vi "Sound-Beeper.vi"() -> (15 "error out":errorcluster)   [LabVIEW 2020]
uses:
  <vilib>/sound2/lvsound2.llb/Sampling Mode.ctl
  <vilib>/sound2/lvsound2.llb/Sound Data Format.ctl
  Math VIs/LinSpace (x0-dx-npts).vi
  <vilib>/sound2/lvsound2.llb/Sound Output Write (DBL Single).vi
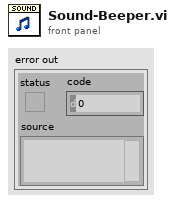
[diagram p1: front panel]
types:
  T1 = typedef "Sound Data Format.ctl" = cluster{"sample rate (S/s)":dbl, "number of channels":i32, "bits per sample":i32}
  T2 = typedef "Sampling Mode.ctl" = i32
  T3 = typedef "Sound Output Task ID.ctl" = u32
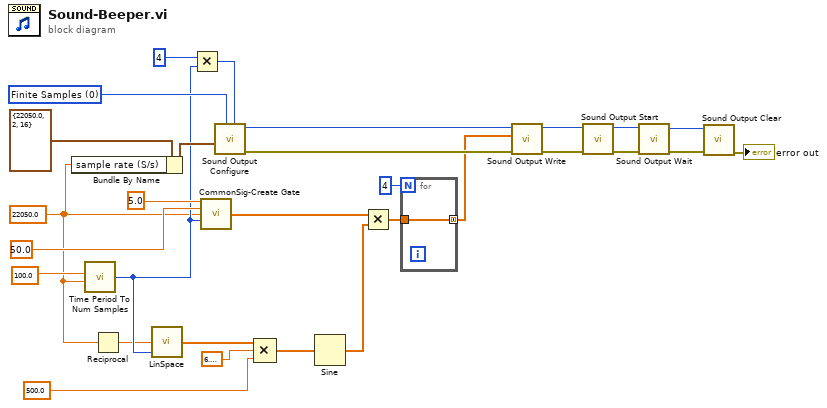
[diagram p0: block diagram]
diagram:
  w11 = 22050.0 ("sample rate (S/s)")
  w29 = T2 0 items=["Finite Samples", "Continuous Samples"] ("sample mode")
  n1 = Bundle By Name(cluster=T1 {"sample rate (S/s)"=22050.0, "number of channels"=2, "bits per sample"=16} ("sound format"), "sample rate (S/s)"=w11) -> (w27:T1)
  n2 = call "Time Period To Num Samples.vi"("Duration (ms)"=100.0 ("sample rate (S/s)"), "Sampling rate (Hz)"=w11) -> ("Samples"=w13:i32)  [unwired: 5 in]
  n3 = Reciprocal(x=w11) -> (1/x=w12:dbl)
  n4 = call-poly "LinSpace.vi"("npts"=w13, "dx"=w12) -> ("Array"=w10:dbl[])  [unwired: 2 in, 1 out]
  n5 = Multiply(x=4, y=w13) -> (x*y=w14:i32)
  n6 = call "CommonSig-Create Gate.vi"("Ramp (ms)"=5.0 ("Duration (ms)"), "Duration (ms)"=50.0 ("sample rate (S/s)"), "Sampling Rate (Hz)"=w11, "Npts"=w13) -> ("Gate"=w6:dbl[])  [unwired: 10 in, 1 out]
  n7 = call <vilib>:"Sound Output Configure.vi"("number of samples/ch"=w14, "sample mode"=w29, "sound format"=w27) -> ("error out"=w23:errorcluster, "task ID"=w24:T3)  [unwired: 7 in]
  n8 = Compound Arithmetic op=MULTIPLY(w10, 6.283185307179586, 500.0) -> (w7:dbl[])
  n9 = Sine(x=w7) -> (sin(x)=w5:dbl[])
  n10 = Multiply(x=w6, y=w5) -> (x*y=w4:dbl[])
  n11 = for {
    N: 4 -> [_]
    tunnel: w4 -> [w30]
    tunnel: [w30] -> w2 mode=concatenating
  }
  n12 = call-poly <vilib>:"Sound Output Write.vi"("error in (no error)"=w23, "data"=w2, "task ID"=w24) -> ("error out"=w21:errorcluster, "task ID out"=w22:T3)  [unwired: 7 in]
  n13 = call <vilib>:"Sound Output Start.vi"("error in (no error)"=w21, "task ID"=w22) -> ("error out"=w20:errorcluster, "task ID out"=w19:T3)  [unwired: 8 in]
  n14 = call <vilib>:"Sound Output Wait.vi"("error in (no error)"=w20, "task ID"=w19) -> ("error out"=w17:errorcluster, "task ID out"=w18:T3)  [unwired: 8 in]
  n15 = call <vilib>:"Sound Output Clear.vi"("error in (no error)"=w17, "task ID"=w18) -> ("error out"=→"error out":errorcluster)  [unwired: 9 in]
